vi "KH TURCK ETHERNETIP RFID WriteTag.vi"(8 "Modul Nr":i32, 11 "TagNr":enum16{"Tag 0", "Tag 1"}(ring)) -> ()   [LabVIEW 2017]
doc: "Write the RFID tag"
uses:
  KH TURCK ETHERNETIP TDef Enum RFID User Command.ctl
  KH TURCK ETHERNETIP RFID Global.vi
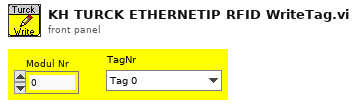
[diagram p1: front panel]
types:
  T1 = typedef "KH TURCK ETHERNETIP TDef Enum RFID User Command.ctl" = enum16{"read", "write", "idle", "inventory"}
  T2 = typedef "KH TURCK ETHERNETIP TDefCluster TURCK RFID.ctl" = cluster{"NumberOfBytes":i32, "State":string, "Counter":i32, "ReadData":u8[], "AnzahlFragmente":i32, "WritingFinished":bool, "ReadingFinished":bool, "UID":u8[], "ActCommand":T3, "SizeFragmentRead":i32, "LengthUID":u16, "WriteDataInclUID":u8[], "Timeout":bool, "SizeFragmentWrite":i32}
  T3 = typedef "KH TURCK ETHERNETIP TDef Enum RFID Act Command.ctl" = enum16{"read", "write", "idle", "Inventory", ""}
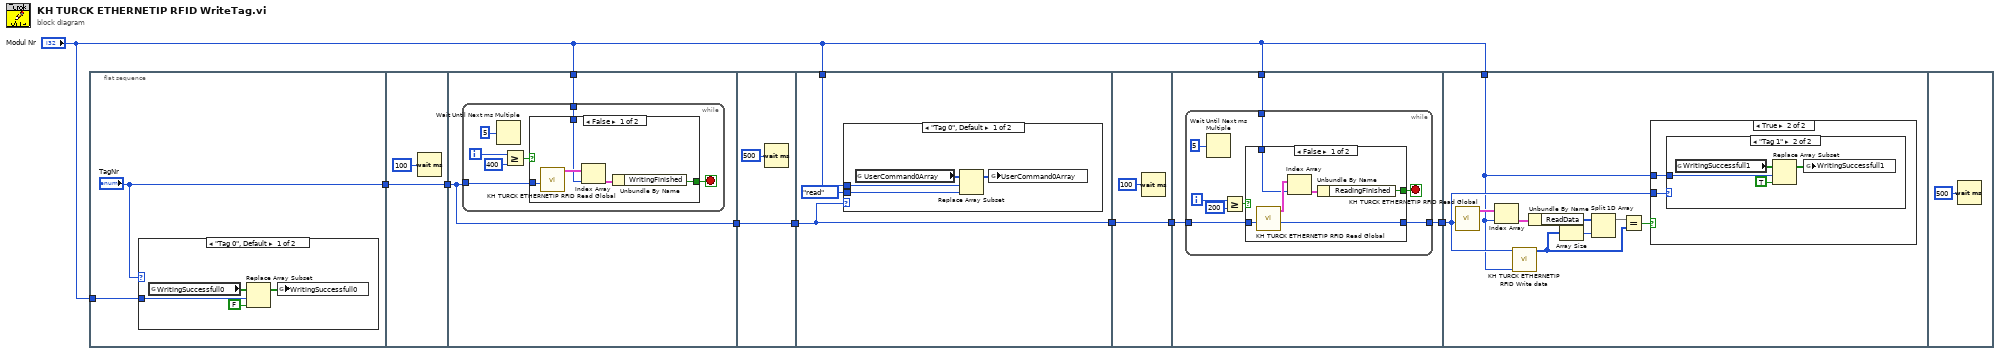
[diagram p0: block diagram]
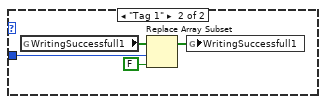
[diagram p2: hidden frame]
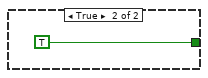
[diagram p3: hidden frame]
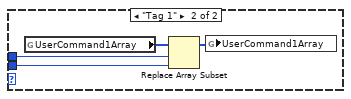
[diagram p4: hidden frame]
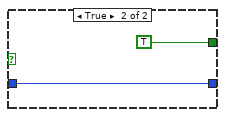
[diagram p5: hidden frame]
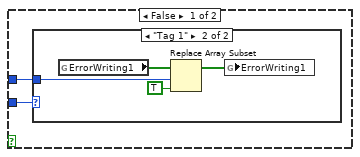
[diagram p6: hidden frame]
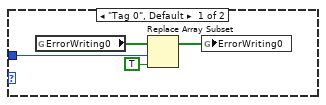
[diagram p7: hidden frame]
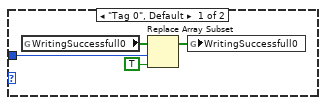
[diagram p8: hidden frame]
diagram:
  n1 = flat-sequence {
    tunnel: ["TagNr"] -> w6
    tunnel: "Modul Nr" -> [w9]
    tunnel: w6 -> [w20]
    tunnel: [w20] -> w5
    tunnel: w5 -> [w22]
    tunnel: [w22] -> w8
    tunnel: "Modul Nr" -> [w21]
    tunnel: w8 -> [w37]
    tunnel: [w37] -> w2
    tunnel: [w40] -> w4
    tunnel: w2 -> [w40]
    tunnel: "Modul Nr" -> [w38]
    tunnel: w4 -> [w50]
    tunnel: [w50] -> w3
    tunnel: w3 -> [w53]
    tunnel: [w52] -> w7
    tunnel: "Modul Nr" -> [w51]
    tunnel: w7 -> [w71]
    tunnel: "Modul Nr" -> [w70]
    frame #0 {
      n2 = case shown="\"Tag 0\", Default" "TagNr" {
        tunnel: w9 -> [w11 w15]
        frame "Tag 0", Default {
          n3 = global read "KH TURCK ETHERNETIP RFID Global.vi" "WritingSuccessfull0"() -> (w14:bool[])
          n4 = Replace Array Subset(array=w14, new element=FALSE ("WritingSuccesfull1"), index=w11) -> (w13:bool[])
          n5 = global write "KH TURCK ETHERNETIP RFID Global.vi" "WritingSuccessfull0"(w13) -> ()
        }
        frame "Tag 1" {
          n6 = global read "KH TURCK ETHERNETIP RFID Global.vi" "WritingSuccessfull1"() -> (w18:bool[])
          n7 = Replace Array Subset(array=w18, new element=FALSE ("WritingSuccesfull1"), index=w15) -> (w17:bool[])
          n8 = global write "KH TURCK ETHERNETIP RFID Global.vi" "WritingSuccessfull1"(w17) -> ()
        }
      }
    }
    frame #1 {
      n9 = Wait (ms)(milliseconds to wait=u32 100) -> ()  [unwired: 1 out]
    }
    frame #2 {
      n10 = while {
        tunnel: w22 -> [w24]
        tunnel: w21 -> [w23]
        i -> [w27]
        stop <- w29 stop-if-true
        n11 = Wait Until Next ms Multiple(millisecond multiple=u32 5) -> ()  [unwired: 1 out]
        n12 = Greater Or Equal?(x=w27, y=400) -> (x >= y?=w25:bool)
        n13 = case shown="False" w25 {
          tunnel: [w34 TRUE ("TimeoutWriting")] -> w29
          tunnel: w24 -> [w33 _]
          tunnel: w23 -> [w31 _]
          frame False {
            n14 = call "KH TURCK ETHERNETIP RFID Read Global.vi"("TagNrIn"=w33) -> ("RFID_GlobalIn"=w32:T2[])  [unwired: 9 in, 1 out]
            n15 = Index Array(array=w32, index=w31) -> (element=w30:T2)
            n16 = Unbundle By Name(w30) -> ("WritingFinished"=w34:bool)
          }
          frame True {
          }
        }
      }
    }
    frame #3 {
      n17 = Wait (ms)(milliseconds to wait=u32 500) -> ()  [unwired: 1 out]
    }
    frame #4 {
      n18 = case shown="\"Tag 0\", Default" w40 {
        tunnel: KH_TURCK_ETHERNETIP_TDef_Enum_RFID_User_Command."read" ("UserCommand") -> [w43 w46]
        tunnel: w38 -> [w41 w45]
        frame "Tag 0", Default {
          n19 = global read "KH TURCK ETHERNETIP RFID Global.vi" "UserCommand0Array"() -> (w44:T1[])
          n20 = Replace Array Subset(array=w44, new element=w43, index=w41) -> (w42:T1[])
          n21 = global write "KH TURCK ETHERNETIP RFID Global.vi" "UserCommand0Array"(w42) -> ()
        }
        frame "Tag 1" {
          n22 = global read "KH TURCK ETHERNETIP RFID Global.vi" "UserCommand1Array"() -> (w48:T1[])
          n23 = Replace Array Subset(array=w48, new element=w46, index=w45) -> (w47:T1[])
          n24 = global write "KH TURCK ETHERNETIP RFID Global.vi" "UserCommand1Array"(w47) -> ()
        }
      }
    }
    frame #5 {
      n25 = Wait (ms)(milliseconds to wait=u32 100) -> ()  [unwired: 1 out]
    }
    frame #6 {
      n26 = while {
        tunnel: w53 -> [w56]
        tunnel: [w55] -> w52
        tunnel: w51 -> [w54]
        i -> [w59]
        stop <- w61 stop-if-true
        n27 = Wait Until Next ms Multiple(millisecond multiple=u32 5) -> ()  [unwired: 1 out]
        n28 = Greater Or Equal?(x=w59, y=200) -> (x >= y?=w57:bool)
        n29 = case shown="False" w57 {
          tunnel: [w67 TRUE ("TimeoutWriting")] -> w61
          tunnel: w56 -> [w66 w68]
          tunnel: [w65 w68] -> w55
          tunnel: w54 -> [w62 _]
          frame False {
            n30 = call "KH TURCK ETHERNETIP RFID Read Global.vi"("TagNrIn"=w66) -> ("TagNrOut"=w65:enum16{"Tag 0", "Tag 1"}, "RFID_GlobalIn"=w64:T2[])  [unwired: 9 in]
            n31 = Index Array(array=w64, index=w62) -> (element=w63:T2)
            n32 = Unbundle By Name(w63) -> ("ReadingFinished"=w67:bool)
          }
          frame True {
          }
        }
      }
    }
    frame #7 {
      n33 = call "KH TURCK ETHERNETIP RFID Read Global.vi"("TagNrIn"=w71) -> ("RFID_GlobalIn"=w73:T2[])  [unwired: 9 in, 1 out]
      n34 = Index Array(array=w73, index=w70) -> (element=w74:T2)
      n35 = call "KH TURCK ETHERNETIP RFID Write data.vi"("Nr RFID"=w70, "Channel"=w71) -> ("Write Data"=w72:u8[])  [unwired: 9 in]
      n36 = Unbundle By Name(w74) -> ("ReadData"=w76:u8[])
      n37 = Array Size(array=w72) -> (size(s)=w78:i32)
      n38 = Split 1D Array(array=w76, index=w78) -> (first subarray=w75:u8[])  [unwired: 1 out]
      n39 = Equal?(x=w75, y=w72) -> (x = y?=w77:bool)
      n40 = case shown="True" w77 {
        tunnel: w71 -> [w80 w90]
        tunnel: w70 -> [w79 w89]
        frame False {
          n41 = case shown="\"Tag 1\"" w80 {
            tunnel: w79 -> [w81 w85]
            frame "Tag 0", Default {
              n42 = global read "KH TURCK ETHERNETIP RFID Global.vi" "ErrorWriting0"() -> (w84:bool[])
              n43 = Replace Array Subset(array=w84, new element=TRUE ("WritingSuccesfull1"), index=w81) -> (w83:bool[])
              n44 = global write "KH TURCK ETHERNETIP RFID Global.vi" "ErrorWriting0"(w83) -> ()
            }
            frame "Tag 1" {
              n45 = global read "KH TURCK ETHERNETIP RFID Global.vi" "ErrorWriting1"() -> (w88:bool[])
              n46 = Replace Array Subset(array=w88, new element=TRUE ("WritingSuccesfull1"), index=w85) -> (w87:bool[])
              n47 = global write "KH TURCK ETHERNETIP RFID Global.vi" "ErrorWriting1"(w87) -> ()
            }
          }
        }
        frame True {
          n48 = case shown="\"Tag 1\"" w90 {
            tunnel: w89 -> [w91 w95]
            frame "Tag 0", Default {
              n49 = global read "KH TURCK ETHERNETIP RFID Global.vi" "WritingSuccessfull0"() -> (w94:bool[])
              n50 = Replace Array Subset(array=w94, new element=TRUE ("WritingSuccesfull1"), index=w91) -> (w93:bool[])
              n51 = global write "KH TURCK ETHERNETIP RFID Global.vi" "WritingSuccessfull0"(w93) -> ()
            }
            frame "Tag 1" {
              n52 = global read "KH TURCK ETHERNETIP RFID Global.vi" "WritingSuccessfull1"() -> (w98:bool[])
              n53 = Replace Array Subset(array=w98, new element=TRUE ("WritingSuccesfull1"), index=w95) -> (w97:bool[])
              n54 = global write "KH TURCK ETHERNETIP RFID Global.vi" "WritingSuccessfull1"(w97) -> ()
            }
          }
        }
      }
    }
    frame #8 {
      n55 = Wait (ms)(milliseconds to wait=u32 500) -> ()  [unwired: 1 out]
    }
  }
